vi "ManualControlASICSUM.vi"() -> ()   [LabVIEW 2012]
uses:
  <vilib>/Utility/NIReport.llb/NI_report.lvclass
  <vilib>/Utility/NIReport.llb/HTML/NI_HTML.lvclass
panel:
  in  "Sum/Maj":bool=TRUE
  in  "stop":bool
  in  "Channel Enable":i32(slide) scale=0.0..6.0
  in  "Attenuation Select":i32(slide) scale=0.0..15.0
  in  "Clipping Select":i32(slide)=3 scale=1.0..3.0
  in  "Ib Clip select":i32(slide)=63 scale=0.0..63.0
  in  "Instrument VISA in":T1={"AWG VISA"="AgilentGenerator1", "Oscilloscope  VISA "="AgilentOsciloscope", "Integration Board IP"="172.16.17.47", "connection ID"=refnum, "report out"=refnum, "report file path"=path "C:/Documents and Settings/CTA_LAB01/Desktop/L0_Asic/L0 Asic Test Data"}
  out "error out":errorcluster
  in  "error in":errorcluster
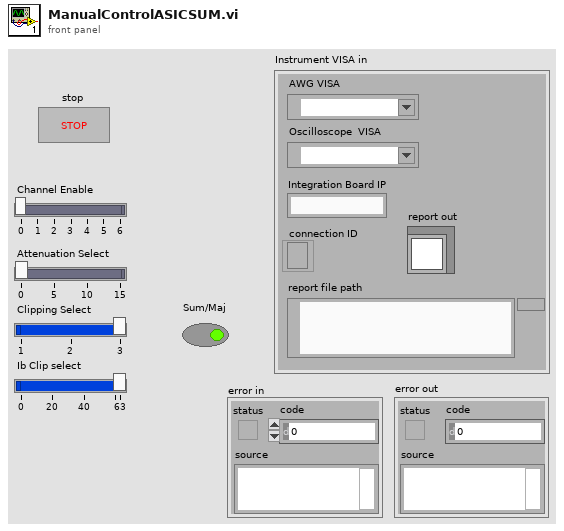
[diagram p1: front panel]
types:
  T1 = cluster{"AWG VISA":refnum<visa-resource-name>, "Oscilloscope  VISA ":refnum<visa-resource-name>, "Integration Board IP":string, "connection ID":refnum<k5>, "report out":refnum<class "NI_report.lvclass">, "report file path":path}
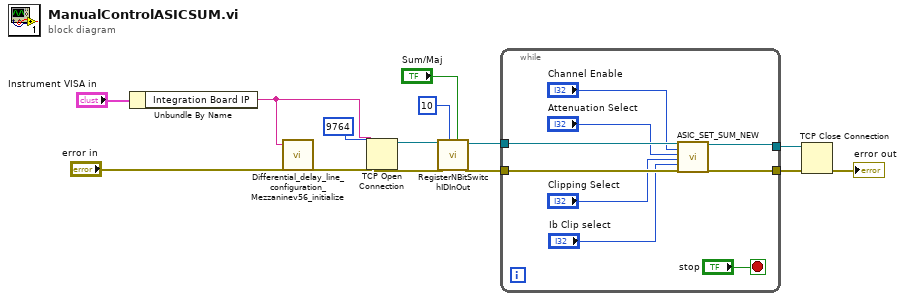
[diagram p0: block diagram]
diagram:
  n1 = Unbundle By Name("Instrument VISA in") -> ("Integration Board IP"=w9:string)
  n2 = call "Differential_delay_line_configuration_Mezzaninev56_initialize.vi"("error in (no error)"="error in", "address"=w9) -> ("error out 2"=w11:errorcluster)  [unwired: 1 in]
  n3 = TCP Open Connection(address=w9, remote port or service name=9764, error in (no error)=w11) -> (connection ID=w2:refnum<k5>, error out=w5:errorcluster)  [unwired: 2 in]
  n4 = call "RegisterNBitSwitchIDInOut.vi"("Switch Bit"="Sum/Maj", "N Bit"=10, "error in (no error)"=w5, "connection ID"=w2) -> ("error out"=w4:errorcluster, "connection ID out"=w3:refnum<k5>)  [unwired: 5 in]
  n5 = while {
    tunnel: [w19] -> w10
    tunnel: w4 -> [w22]
    tunnel: w3 -> [w20]
    tunnel: [w21] -> w1
    stop <- "stop" stop-if-true
    n6 = call "ASIC_SET_SUM_NEW.vi"("connection ID"=w20, "Channel Enable"="Channel Enable", "Attenuation Select"="Attenuation Select", "Clipping Select"="Clipping Select", "Ib Clip select"="Ib Clip select", "error in"=w22) -> ("connection ID out"=w19:refnum<k5>, "error out"=w21:errorcluster)  [unwired: 12 in]
  }
  n7 = TCP Close Connection(connection ID=w10, error in (no error)=w1) -> (error out=→"error out":errorcluster)  [unwired: 1 in, 1 out]
